vi "Update Round.vi"(8 "error in (no error)":errorcluster, 10 "Round":u32, 11 "Dashboard Panel in":refnum<class "Dashboard Panel.lvclass">) -> (0 "error out":errorcluster, 3 "Dashboard Panel out":refnum<class "Dashboard Panel.lvclass">)   [LabVIEW 2020, in "SB App.lvlib" / "Dashboard Panel.lvclass"]
uses:
  Dashboard Panel.lvclass
  Dashboard Panel.lvclass/Dashboard Panel.ctl
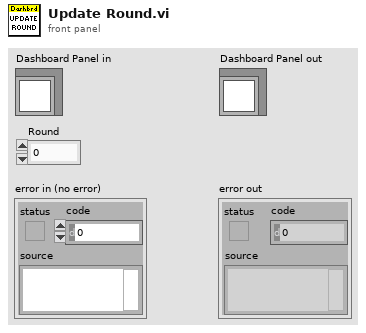
[diagram p1: front panel]
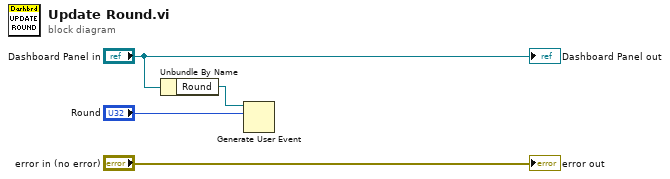
[diagram p0: block diagram]
diagram:
  n1 = Unbundle By Name("Dashboard Panel in") -> ("Round"=w2:refnum<user-event>)
  n2 = Generate User Event(user event=w2, event data cluster="Round") -> ()  [unwired: 2 in, 2 out]
  "error out" <- "error in (no error)"
  "Dashboard Panel out" <- "Dashboard Panel in"
